vi "NI 9205 Gen Configuration (Host).vi"(1 "Gen Type":enum8{"Gen AI", "Gen DI", "Gen DO"}(ring), 3 "AI Channel and Settings":T3 {"AI Channel" max=31}, 5 "DO Data":bool) -> (16 "IO Sample\nConfiguration":u16=10296 format="%x")   [LabVIEW 2013]
uses:
  <vilib>/LabVIEW Targets/FPGA/cRIO/shared/nicrio_ModuleControls/nicrio_cRIO-9205_VoltageRange.ctl
  <vilib>/LabVIEW Targets/FPGA/cRIO/shared/nicrio_ModuleControls/nicrio_cRIO-9205_TerminalMode.ctl
panel:
  out "Numeric 2":u16=10296 format="%016d"
  out "Numeric":u16=10296 format="%016b"
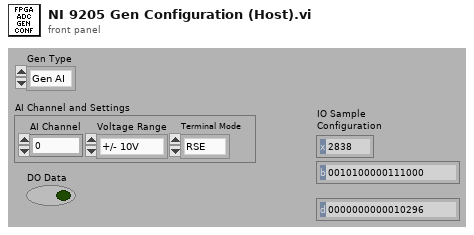
[diagram p1: front panel]
types:
  T1 = typedef "nicrio_cRIO-9205_VoltageRange.ctl" = enum8{"+/- 10V", "+/- 5V", "+/- 1V", "+/- 200mV"}
  T2 = typedef "nicrio_cRIO-9205_TerminalMode.ctl" = enum8{"RSE", "NRSE", "DIFF"}
  T3 = cluster{"AI Channel":u8, "Voltage Range":T1, "Terminal Mode":T2}
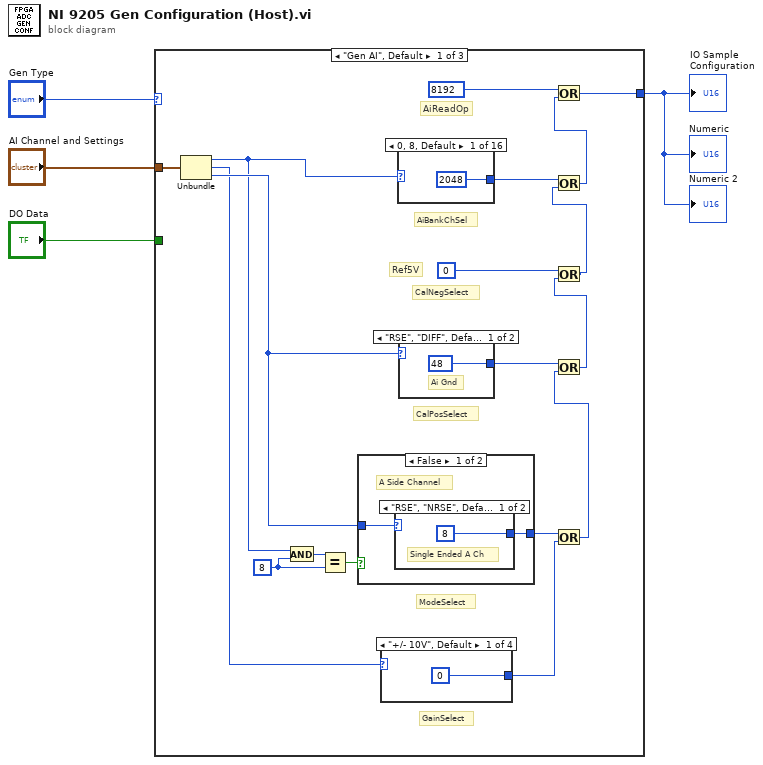
[diagram p0: block diagram]
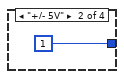
[diagram p2: hidden frame]
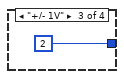
[diagram p3: hidden frame]
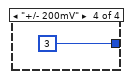
[diagram p4: hidden frame]
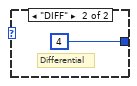
[diagram p5: hidden frame]
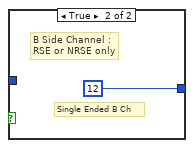
[diagram p6: hidden frame]
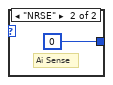
[diagram p7: hidden frame]
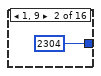
[diagram p8: hidden frame]
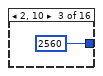
[diagram p9: hidden frame]
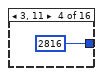
[diagram p10: hidden frame]
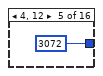
[diagram p11: hidden frame]
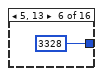
[diagram p12: hidden frame]
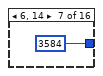
[diagram p13: hidden frame]
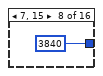
[diagram p14: hidden frame]
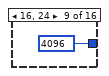
[diagram p15: hidden frame]
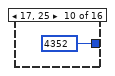
[diagram p16: hidden frame]
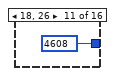
[diagram p17: hidden frame]
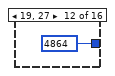
[diagram p18: hidden frame]
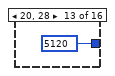
[diagram p19: hidden frame]
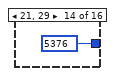
[diagram p20: hidden frame]
diagram:
  n1 = case shown="\"Gen AI\", Default" "Gen Type" {
    tunnel: "DO Data" -> [_ _ w55]
    tunnel: [w8 u16 0 w51] -> w1
    tunnel: "AI Channel and Settings" -> [w22 _ _]
    frame "Gen AI", Default {
      w20 = u8 8 ("y")
      # "GainSelect"
      # "ModeSelect"
      # "Ref5V"
      # "CalNegSelect"
      # "CalPosSelect"
      # "AiReadOp"
      # "AiBankChSel"
      n2 = Unbundle(w22) -> ("AI Channel"=w16:u8, "Voltage Range"=w17:T1, "Terminal Mode"=w18:T2)
      n3 = And(x=w16, y=w20) -> (x .and. y?=w21:u8)
      n4 = Equal?(x=w21, y=w20) -> (x = y?=w19:bool)
      n5 = case shown="False" w19 {
        tunnel: w18 -> [w28 _]
        tunnel: [w27 u16 12] -> w11
        frame False {
          # "A Side Channel"
          n6 = case shown="\"RSE\", \"NRSE\", Default" w28 {
            tunnel: [u16 8 u16 4] -> w27
            frame "RSE", "NRSE", Default {
              # "Single Ended A Ch"
            }
            frame "DIFF" {
              # "Differential"
            }
          }
        }
        frame True {
          # "Single Ended B Ch"
          # "B Side Channel :\nRSE or NRSE only"
        }
      }
      n7 = case shown="\"+/- 10V\", Default" w17 {
        tunnel: [u16 0 u16 1 u16 2 u16 3] -> w12
        frame "+/- 10V", Default {
        }
        frame "+/- 5V" {
        }
        frame "+/- 1V" {
        }
        frame "+/- 200mV" {
        }
      }
      n8 = case shown="0, 8, Default" w16 {
        tunnel: [u16 2048 u16 2304 u16 2560 u16 2816 u16 3072 u16 3328 u16 3584 u16 3840 u16 4096 u16 4352 u16 4608 u16 4864 u16 5120 u16 5376 u16 5632 u16 5888] -> w14
        frame 0, 8, Default {
        }
        frame 1, 9 {
        }
        frame 2, 10 {
        }
        frame 3, 11 {
        }
        frame 4, 12 {
        }
        frame 5, 13 {
        }
        frame 6, 14 {
        }
        frame 7, 15 {
        }
        frame 16, 24 {
        }
        frame 17, 25 {
        }
        frame 18, 26 {
        }
        frame 19, 27 {
        }
        frame 20, 28 {
        }
        frame 21, 29 {
        }
        frame 22, 30 {
        }
        frame 23, 31 {
        }
      }
      n9 = case shown="\"RSE\", \"DIFF\", Default" w18 {
        tunnel: [u16 48 u16 0] -> w13
        frame "RSE", "DIFF", Default {
          # "Ai Gnd"
        }
        frame "NRSE" {
          # "Ai Sense"
        }
      }
      n10 = Or(x=w11, y=w12) -> (x .or. y?=w10:u16)
      n11 = Or(x=w13, y=w10) -> (x .or. y?=w6:u16)
      n12 = Or(x=u16 0, y=w6) -> (x .or. y?=w5:u16)
      n13 = Or(x=w14, y=w5) -> (x .or. y?=w9:u16)
      n14 = Or(x=u16 8192, y=w9) -> (x .or. y?=w8:u16)
    }
    frame "Gen DI" {
      # "Read DI"
    }
    frame "Gen DO" {
      # "Write DO"
      n15 = Boolean To (0,1)(Boolean=w55) -> (0, 1=w53:i16)
      n16 = To Unsigned Word Integer(number=w53) -> (unsigned 16bit integer=w52:u16)
      n17 = Or(x=u16 16384, y=w52) -> (x .or. y?=w51:u16)
    }
  }
  "IO Sample\nConfiguration" <- w1
  "Numeric" <- w1
  "Numeric 2" <- w1
